vi "ExposeSetRefnumVariantValue.vi"(8 "Value":variant, 10 "Control":variant, 11 "Value In (reference)":refnum<data-value>) -> (0 "IsControl":bool)   [LabVIEW 2017]
panel:
  out "Control":refnum<vi>
  out "Control being updated":string
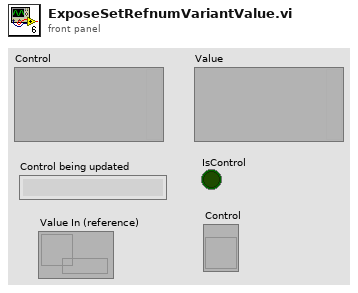
[diagram p1: front panel]
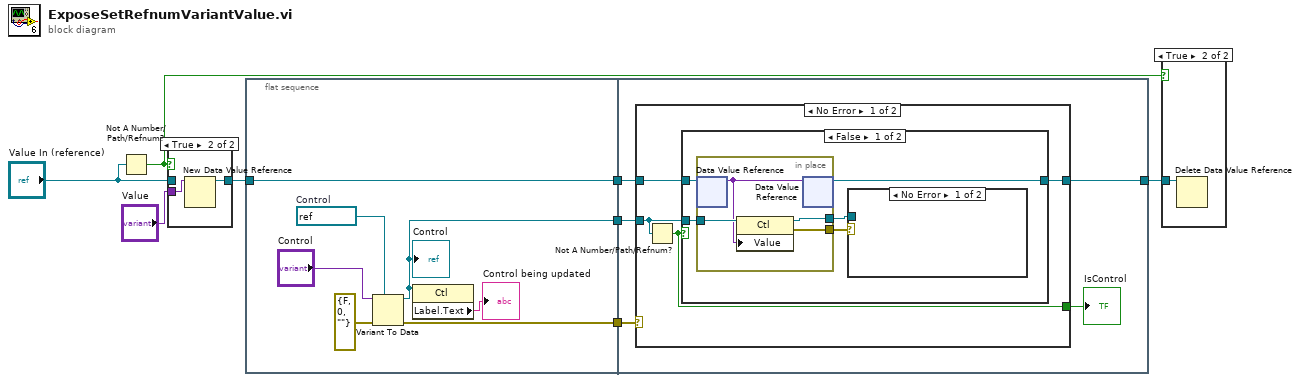
[diagram p0: block diagram]
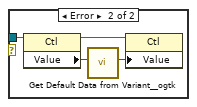
[diagram p4: hidden frame]
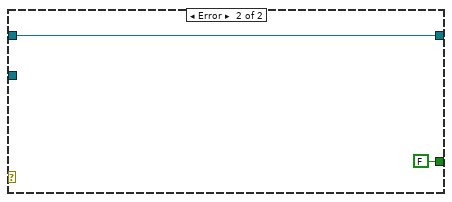
[diagram p6: hidden frame]
diagram:
  n1 = Not A Number/Path/Refnum?(number/path/refnum="Value In (reference)") -> (NaN/Path/Refnum?=w2:bool)
  n2 = case shown="True" w2 {
    tunnel: "Value" -> [_ w11]
    tunnel: "Value In (reference)" -> [w9 _]
    tunnel: [w9 w10] -> w4
    frame False {
    }
    frame True {
      n3 = New Data Value Reference(data value=w11) -> (data value reference=w10:refnum<data-value>)  [unwired: 1 in, 1 out]
    }
  }
  n4 = flat-sequence {
    tunnel: [w15] -> w8
    tunnel: [w14] -> w7
    tunnel: w4 -> [w12]
    tunnel: [w12] -> w3
    tunnel: w8 -> [w22]
    tunnel: w7 -> [w21]
    tunnel: w3 -> [w20]
    tunnel: [w19] -> w1
    frame #0 {
      w18 = refnum<vi> refnum  # Control
      n5 = Variant To Data(error in=errorcluster {"status"=FALSE, "code"=0, "source"=""}, type=w18, Variant="Control") -> (data=w14:refnum<vi>, error out=w15:errorcluster)
      "Control" <- w14
      n6 = property class="Ctl"(reference=w14) -> ("Label.Text"=→"Control being updated":string)  [unwired: 1 in, 2 out]
    }
    frame #1 {
      n7 = case shown="No Error" w22 {
        tunnel: w21 -> [w27 _]
        tunnel: [w26 FALSE] -> w23
        tunnel: w20 -> [w25 w42]
        tunnel: [w24 w42] -> w19
        frame No Error {
          n8 = Not A Number/Path/Refnum?(number/path/refnum=w27) -> (NaN/Path/Refnum?=w26:bool)
          n9 = case shown="False" w26 {
            tunnel: w27 -> [w32 _]
            tunnel: w25 -> [w29 w41]
            tunnel: [w28 w41] -> w24
            frame False {
              n10 = in-place {
                in-place-border: w32 -> [w36]
                in-place-border: [w35] -> w31
                in-place-border: [w34] -> w30
                n11 = in-place-dvr #1(w29) -> (w33:variant)  [unwired: 1 out]
                n12 = property class="Ctl"(reference=w36, "Value"=w33) -> (reference out=w34:refnum<vi>, error out=w35:errorcluster)  [unwired: 1 in]
                n13 = in-place-dvr #1(w33) -> (w28:refnum<data-value>)  [unwired: 1 out]
              }
              n14 = case shown="No Error" w31 {
                tunnel: w30 -> [_ w40]
                frame No Error {
                }
                frame Error {
                  n15 = property class="Ctl"(reference=w40) -> (reference out=w37:refnum<vi>, "Value"=w39:variant)  [unwired: 1 in, 1 out]
                  n16 = call <userlib>:"Get Default Data from Variant__ogtk.vi"("Variant"=w39) -> ("Default VData"=w38:variant)  [unwired: 9 in, 1 out]
                  n17 = property class="Ctl"(reference=w37, "Value"=w38) -> ()  [unwired: 1 in, 2 out]
                }
              }
            }
            frame True {
            }
          }
        }
        frame Error {
        }
      }
      "IsControl" <- w23
    }
  }
  n18 = case shown="True" w2 {
    tunnel: w1 -> [_ w44]
    frame False {
    }
    frame True {
      n19 = Delete Data Value Reference(data value reference=w44) -> ()  [unwired: 1 in, 2 out]
    }
  }
